vi "Inst.FP.GHSmodeStringToEnum.vi"(1 "mode string":string) -> (0 "mode enum":T1)   [LabVIEW 2019, in "Inst.FP.lvclass"]
uses:
  Inst.FP.lvclass
  Typedefs/Inst.FP.Modes--Enum.ctl
  047fb9ee-60f3-42ae-aff5-f45a097b9959.vi
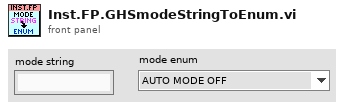
[diagram p1: front panel]
types:
  T1 = typedef "Inst.FP.lvclass/Inst.FP.Modes--Enum.ctl" = enum16{"AUTO MODE OFF", "START", "CONDENSING 3He", "CONDENSING 4He", "NORMAL CIRCULATION", "RECOVERY OF THE MIXTURE", "RECOVERY: BLOCKAGE or OVERPRESSURE"}
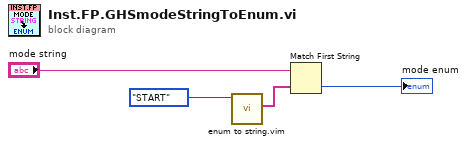
[diagram p0: block diagram]
diagram:
  n1 = call "enum to string.vim"("enum in"=Inst.FP.Modes--Enum."START" ("Mode")) -> ("strings out"=w4:string[])  [unwired: 9 in, 1 out]
  n2 = Match First String(2:w4, 3:"mode string") -> (0:→"mode enum":i32)  [unwired: 1 out]
